vi "HandleInput.vi"(8 "error in (no error)":errorcluster, 11 "TeleopInstruction":T1) -> (0 "error out":errorcluster, 2 "SkippedData?":bool, 3 "Time":u32)   [LabVIEW 2013]
uses:
  TeleopInstruction.ctl
  DriveData.ctl
  DoubleSolenoidAction.ctl
  CollectorWrapAction.ctl
  QueueSubsystem.ctl
  QueueAction.ctl
panel:
  in  "Deadzone":dbl=0.1
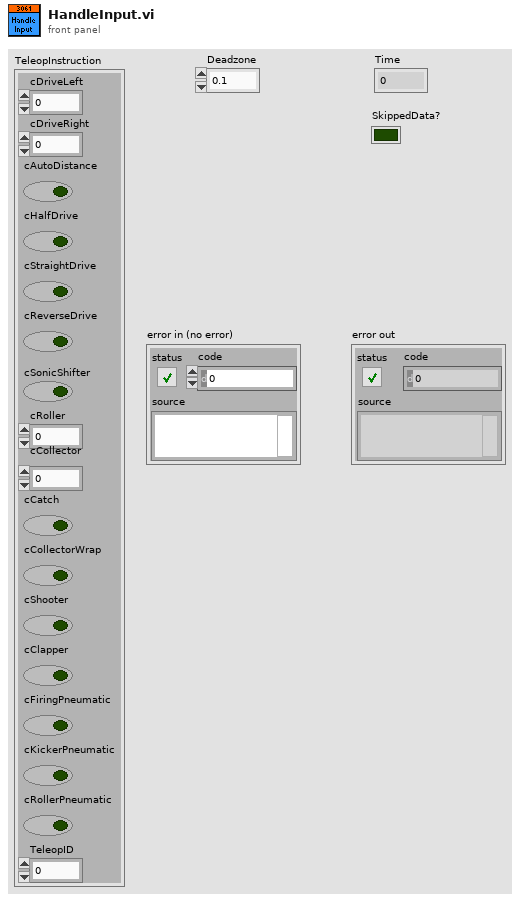
[diagram p1: front panel]
types:
  T1 = typedef "TeleopInstruction.ctl" = cluster{"cDriveLeft":dbl, "cDriveRight":dbl, "cAutoDistance":bool, "cHalfDrive":bool, "cStraightDrive":bool, "cReverseDrive":bool, "cSonicShifter":bool, "cRoller":dbl, "cCollector":dbl, "cCatch":bool, "cCollectorWrap":bool, "cShooter":bool, "cClapper":bool, "cFiringPneumatic":bool, "cKickerPneumatic":bool, "cRollerPneumatic":bool, "TeleopID":i32}
  T2 = typedef "CollectorWrapAction.ctl" = enum16{"PreCollect", "Collect", "Stop"}
  T3 = typedef "DoubleSolenoidAction.ctl" = enum16{"Init", "Middle", "In", "Out"}
  T4 = typedef "DriveData.ctl" = cluster{"cDriveLeft":dbl, "cDriveRight":dbl, "cHalfDrive":bool, "cStraightDrive":bool, "cReverseDrive":bool}
  T5 = typedef "RollerAction.ctl" = enum16{"Init", "Off", "Forward", "Reverse"}
  T6 = typedef "QueueAction.ctl" = enum16{"Init", "SetValue", "Disable"}
  T7 = typedef "QueueSubsystem.ctl" = enum16{"Drive", "SonicShifter", "Kicker", "FiringPneumatic", "RollerPneumatic", "Clapper", "RollerMotor", "CollectorMotor"}
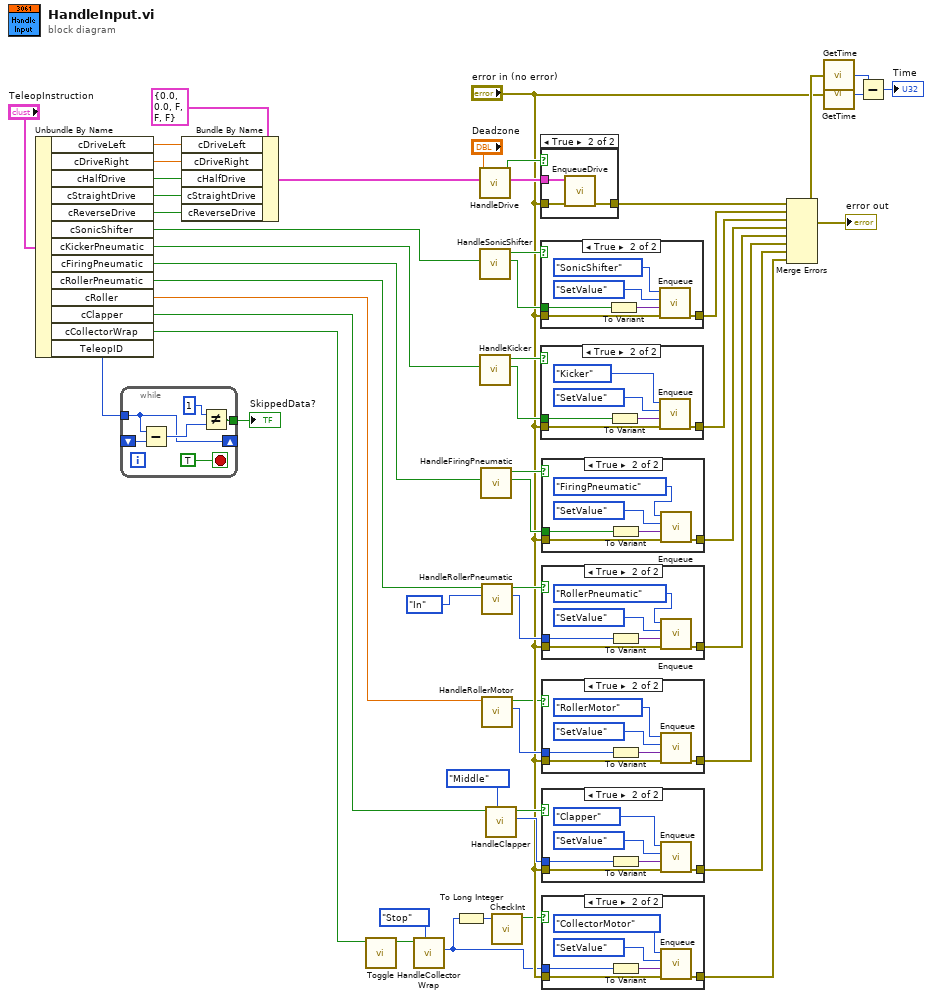
[diagram p0: block diagram]
diagram:
  n1 = Unbundle By Name("TeleopInstruction") -> ("cDriveLeft"=w42:dbl, "cDriveRight"=w41:dbl, "cHalfDrive"=w45:bool, "cStraightDrive"=w44:bool, "cReverseDrive"=w43:bool, "cSonicShifter"=w34:bool, "cKickerPneumatic"=w32:bool, "cFiringPneumatic"=w25:bool, "cRollerPneumatic"=w24:bool, "cRoller"=w2:dbl, "cClapper"=w13:bool, "cCollectorWrap"=w7:bool, "TeleopID"=w3:i32)
  n2 = while {
    tunnel: [w54] -> w4
    tunnel: w3 -> [w53]
    shift-right: [w53] -> _
    shift-left: _ -> [w57]
    stop <- TRUE stop-if-true
    n3 = Subtract(x=w53, y=w57) -> (x-y=w56:i32)
    n4 = Not Equal?(x=1, y=w56) -> (x != y?=w54:bool)
  }
  "SkippedData?" <- w4
  n5 = Bundle By Name(cluster=T4 {"cDriveLeft"=0.0, "cDriveRight"=0.0, "cHalfDrive"=FALSE, "cStraightDrive"=FALSE, "cReverseDrive"=FALSE} ("DriveInstruction"), "cDriveLeft"=w42, "cDriveRight"=w41, "cHalfDrive"=w45, "cStraightDrive"=w44, "cReverseDrive"=w43) -> (w39:T4)
  n6 = call "Toggle.vi"("Input"=w7) -> ("Output"=w8:bool)  [unwired: 10 in]
  n7 = call "HandleCollectorWrap.vi"("InitState"=CollectorWrapAction."Stop" ("Action"), "Toggle?"=w8) -> ("State"=w5:T2)  [unwired: 8 in, 1 out]
  n8 = To Long Integer(number=w5) -> (32bit integer=w6:i32)
  n9 = call "HandleDrive.vi"("DriveInstruction"=w39, "Deadzone"="Deadzone") -> ("DriveInstruction"=w40:T4, "Enqueue?"=w47:bool)  [unwired: 8 in]
  n10 = call "HandleSonicShifter.vi"("cSonicShifter"=w34) -> ("Output"=w33:bool, "Enqueue?"=w38:bool)  [unwired: 9 in]
  n11 = call "HandleKicker.vi"("cKicker"=w32) -> ("Output"=w30:bool, "Enqueue?"=w31:bool)  [unwired: 9 in]
  n12 = call "HandleFiringPneumatic.vi"("cFiringPneumatic"=w25) -> ("Output"=w27:bool, "Enqueue?"=w26:bool)  [unwired: 9 in]
  n13 = call "HandleRollerPneumatic.vi"("InitState"=DoubleSolenoidAction."In", "Toggle?"=w24) -> ("State"=w22:T3, "Enqueue?"=w20:bool)  [unwired: 7 in, 1 out]
  n14 = call "HandleRollerMotor.vi"("JoystickValue"=w2) -> ("StateOut"=w19:T5, "Enqueue?"=w1:bool)  [unwired: 8 in, 1 out]
  n15 = call "HandleClapper.vi"("InitState"=DoubleSolenoidAction."Middle", "Toggle?"=w13) -> ("State"=w15:T3, "Enqueue?"=w16:bool)  [unwired: 7 in, 1 out]
  n16 = call "CheckInt.vi"("Integer"=w6) -> ("Changed?"=w9:bool)  [unwired: 10 in]
  n17 = case shown="True" w47 {
    tunnel: [w59 w62] -> w37
    tunnel: "error in (no error)" -> [w59 w61]
    tunnel: w40 -> [_ w60]
    frame False {
    }
    frame True {
      n18 = call "EnqueueDrive.vi"("error in (no error)"=w61, "DriveInstruction"=w60) -> ("error out"=w62:errorcluster)  [unwired: 9 in]
    }
  }
  n19 = case shown="True" w38 {
    tunnel: "error in (no error)" -> [w63 w69]
    tunnel: [w63 w68] -> w36
    tunnel: w33 -> [_ w64]
    frame False {
    }
    frame True {
      n20 = To Variant(anything=w64) -> (Variant=w65:variant)
      n21 = call "Enqueue.vi"("error in (no error)"=w69, "Data"=w65, "Action"=QueueAction."SetValue", "Subsystem"=QueueSubsystem."SonicShifter") -> ("error out"=w68:errorcluster)  [unwired: 7 in]
    }
  }
  n22 = case shown="True" w31 {
    tunnel: w30 -> [_ w72]
    tunnel: "error in (no error)" -> [w70 w76]
    tunnel: [w70 w71] -> w29
    frame False {
    }
    frame True {
      n23 = To Variant(anything=w72) -> (Variant=w73:variant)
      n24 = call "Enqueue.vi"("error in (no error)"=w76, "Data"=w73, "Action"=QueueAction."SetValue", "Subsystem"=QueueSubsystem."Kicker") -> ("error out"=w71:errorcluster)  [unwired: 7 in]
    }
  }
  n25 = case shown="True" w26 {
    tunnel: w27 -> [_ w79]
    tunnel: "error in (no error)" -> [w77 w83]
    tunnel: [w77 w78] -> w28
    frame False {
    }
    frame True {
      n26 = To Variant(anything=w79) -> (Variant=w80:variant)
      n27 = call "Enqueue.vi"("error in (no error)"=w83, "Data"=w80, "Action"=QueueAction."SetValue", "Subsystem"=QueueSubsystem."FiringPneumatic") -> ("error out"=w78:errorcluster)  [unwired: 7 in]
    }
  }
  n28 = case shown="True" w20 {
    tunnel: w22 -> [_ w86]
    tunnel: "error in (no error)" -> [w84 w90]
    tunnel: [w84 w85] -> w21
    frame False {
    }
    frame True {
      n29 = To Variant(anything=w86) -> (Variant=w87:variant)
      n30 = call "Enqueue.vi"("error in (no error)"=w90, "Data"=w87, "Action"=QueueAction."SetValue", "Subsystem"=QueueSubsystem."RollerPneumatic") -> ("error out"=w85:errorcluster)  [unwired: 7 in]
    }
  }
  n31 = case shown="True" w1 {
    tunnel: w19 -> [_ w93]
    tunnel: "error in (no error)" -> [w91 w97]
    tunnel: [w91 w92] -> w18
    frame False {
    }
    frame True {
      n32 = To Variant(anything=w93) -> (Variant=w94:variant)
      n33 = call "Enqueue.vi"("error in (no error)"=w97, "Data"=w94, "Action"=QueueAction."SetValue", "Subsystem"=QueueSubsystem."RollerMotor") -> ("error out"=w92:errorcluster)  [unwired: 7 in]
    }
  }
  n34 = case shown="True" w16 {
    tunnel: w15 -> [_ w100]
    tunnel: "error in (no error)" -> [w98 w104]
    tunnel: [w98 w99] -> w17
    frame False {
    }
    frame True {
      n35 = To Variant(anything=w100) -> (Variant=w101:variant)
      n36 = call "Enqueue.vi"("error in (no error)"=w104, "Data"=w101, "Action"=QueueAction."SetValue", "Subsystem"=QueueSubsystem."Clapper") -> ("error out"=w99:errorcluster)  [unwired: 7 in]
    }
  }
  n37 = case shown="True" w9 {
    tunnel: w5 -> [_ w107]
    tunnel: "error in (no error)" -> [w105 w111]
    tunnel: [w105 w106] -> w11
    frame False {
    }
    frame True {
      n38 = To Variant(anything=w107) -> (Variant=w108:variant)
      n39 = call "Enqueue.vi"("error in (no error)"=w111, "Data"=w108, "Action"=QueueAction."SetValue", "Subsystem"=QueueSubsystem."CollectorMotor") -> ("error out"=w106:errorcluster)  [unwired: 7 in]
    }
  }
  n40 = Merge Errors(w37, w36, w29, w28, w21, w18, w17, w11) -> (w35:errorcluster)
  "error out" <- w35
  n41 = call "GetTime.vi"("error in"=w35) -> ("Time"=w51:u32)
  n42 = call "GetTime.vi"("error in"="error in (no error)") -> ("Time"=w50:u32)
  n43 = Subtract(x=w51, y=w50) -> (x-y=→"Time":u32)
